vi "SeqMgr.Error, Build Function Name Error Message.vi"(8 "error in":errorcluster, 9 "Data2":variant, 10 "Funct_Seq Name":string, 11 "Local Q":refnum<queue>) -> (0 "error out":errorcluster)   [LabVIEW 2024, in "EQMF.lvlib" / "SeqMgr.lvlib"]
uses:
  SeqMgr.lvlib
  Queues/Q.Element.ctl
  Queues/Q.Msg Return Info.ctl
  Event Log/Event Log.lvlib
  Queues/Queue Utils.lvlib
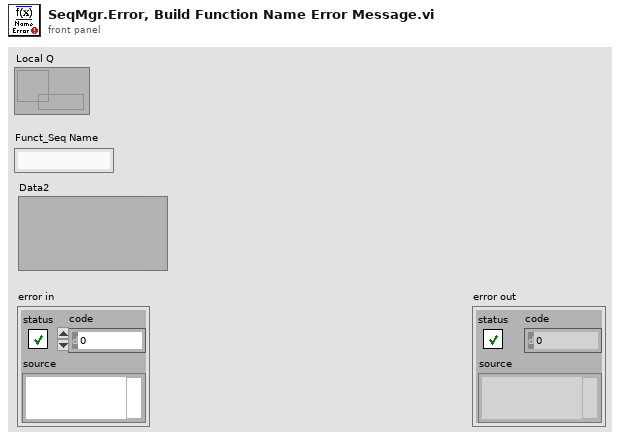
[diagram p1: front panel]
types:
  T1 = typedef "EQMF.lvlib/Queue Utils.lvlib/Q.Msg Return Info.ctl" = cluster{"Ret Q":refnum<queue>, "Ret Msg":T2, "SeqNum":i32}
  T2 = typedef "EQMF.lvlib/Queue Utils.lvlib/Q.Element.ctl" = cluster{"Cmd":string, "Sub":string, "Data1":variant, "Data2":variant}
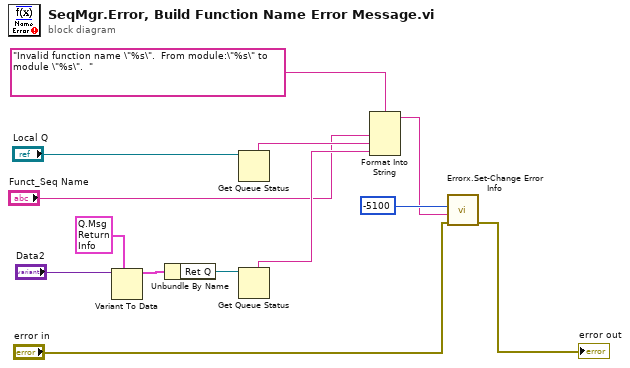
[diagram p0: block diagram]
diagram:
  n1 = Variant To Data(type=T1 {"Ret Q"=refnum, "Ret Msg"={"Cmd"="", "Sub"="", "Data1"=variant, "Data2"=variant}, "SeqNum"=0} ("Cmd Ret Req Data"), Variant="Data2") -> (data=w8:T1)  [unwired: 1 in, 1 out]
  n2 = Unbundle By Name(w8) -> ("Ret Q"=w7:refnum<queue>)
  n3 = Get Queue Status(queue="Local Q") -> (queue name=w11:string)  [unwired: 2 in, 7 out]
  n4 = Get Queue Status(queue=w7) -> (queue name=w6:string)  [unwired: 2 in, 7 out]
  n5 = Format Into String(format string="Invalid function name \"%s\".  From module:\"%s\" to module \"%s\".  ", "Funct_Seq Name", w11, w6) -> (resulting string=w10:string)  [unwired: 2 in, 1 out]
  n6 = call "Errorx.Set-Change Error Info.vi"("error in"="error in", "Description"=w10, "Code(0 = no change)"=-5100) -> ("error out"=→"error out":errorcluster)  [unwired: 8 in]
